vi "All Directions.vi"() -> (3 "All directions":T1[](array[typedef]))   [LabVIEW 2020, in "DS Square.lvlib"]
uses:
  DS Square.lvlib
  Type Defs/Direction Enum.ctl
  Type Defs/SB Type Defs.lvlib
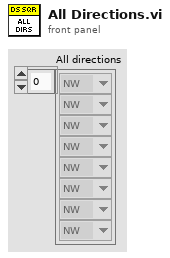
[diagram p1: front panel]
types:
  T1 = typedef "SB Type Defs.lvlib/Direction Enum.ctl" = enum16{"NW", "N", "NE", "E", "SE", "S", "SW", "W"}
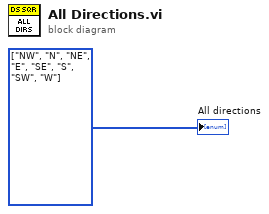
[diagram p0: block diagram]
diagram:
  w1 = T1[] [enum."NW", enum."N", enum."NE", enum."E", enum."SE", enum."S", enum."SW", enum."W"] items=["NW", "N", "NE", "E", "SE", "S", "SW", "W"] ("All directions")
  "All directions" <- w1
